vi "GetDiagramOutputs.vi"(6 "error in":errorcluster, 9 "Structure in":refnum<class "Structure.lvclass">) -> (0 "error out":errorcluster, 3 "Structure out":refnum<class "Structure.lvclass">, 4 "output terminals":refnum<class "Terminal.lvclass">[][](array[class]))   [LabVIEW 2014, in "Raspberry Pi Compatible Compiler for LabVIEW.lvlib" / "Structure.lvclass"]
uses:
  Structure.lvclass
  Terminal/Terminal.lvclass
  Tunnel/Tunnel.lvclass/Tunnel.ctl
  Tunnel/Tunnel.lvclass
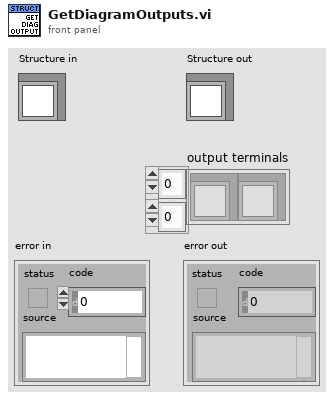
[diagram p1: front panel]
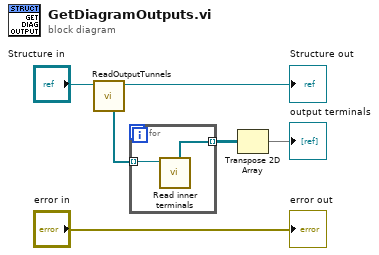
[diagram p0: block diagram]
diagram:
  n1 = call-dynamic "ReadOutputTunnels.vi"("Structure in"="Structure in") -> ("Structure out"=→"Structure out":refnum<class "Structure.lvclass">, "outputs"=w5:refnum<class "Tunnel.lvclass">[])  [unwired: 7 in]
  n2 = for {
    tunnel: w5 -> [w8] mode=indexing
    tunnel: [w7] -> w2 mode=indexing
    n3 = call "Read inner terminals.vi"("Tunnel in"=w8) -> ("inner terminals"=w7:refnum<class "Terminal.lvclass">[])  [unwired: 7 in, 1 out]
  }
  n4 = Transpose 2D Array(2D array=w2) -> (transposed array=→"output terminals":refnum<class "Terminal.lvclass">[][])
  "error out" <- "error in"
